vi "PPG_ABC.ProcCases.vi"(0 "i ref in":refnum<vi>, 1 "selector":string, 2 "Data":T1, 3 "call cluster":T2={"Object"="", "Selector"="", "CallType"=enum."synchronous", "Async Object"="", "Async Selector"="", "Data Descriptor"="", "Data"=[], "Error #"=0, "Expire"=0}, 5 "error in (no error)":errorcluster) -> (14 "i ref out":refnum<vi>, 17 "answer cluster":T2={"Object"="", "Selector"="", "CallType"=enum."synchronous", "Async Object"="", "Async Selector"="", "Data Descriptor"="", "Data"=[], "Error #"=0, "Expire"=0}, 19 "error out":errorcluster)   [LabVIEW 2014, in "PPG_ABC.lvlib"]
doc: "This method is called by a process from within the default case in the event loop. The methods of a class that are linked to events will be called from THIS method. Add your code here."
uses:
  PPG_ABC.lvlib
  CSCore/CSSystem/CoreDefs/CoreDefs.call_type.ctl
  CSCore/BaseProcess/BaseProcess.descriptor string definition.ctl
  CSCore/CSSystem/CoreDefs/CoreDefs.rawDataType.ctl
  CSCore/CSSystem/CoreLib/CoreLib.string 2 byte array.vi
  CSCore/CSSystem/CoreLib/CoreLib.byte array 2 int.vi
  CSCore/CSSystem/CoreLib/CoreLib.int 2 byte array.vi
  CSCore/CSSystem/CoreLib/CoreLib.byte array 2 double.vi
  CSCore/CSSystem/CoreLib/CoreLib.byte array 2 string.vi
  CSCore/CSSystem/CoreLib/CoreLib.lvlib
  CSCore/BaseProcess/BaseProcess.lvlib
  NI_FPGA_PPG/NI_FPGA_PPG.lvlib
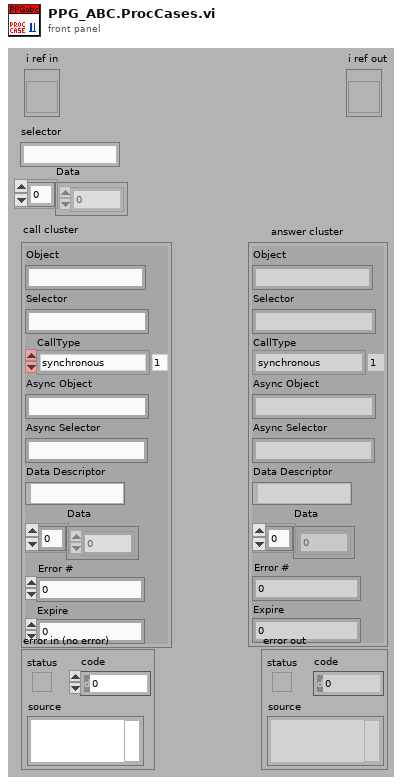
[diagram p1: front panel]
types:
  T1 = typedef "CoreDefs.rawDataType.ctl" = i8[]
  T2 = typedef "CoreDefs.call_type.ctl" = cluster{"Object":string, "Selector":string, "CallType":enum16{"simple", "synchronous", "asynchronous"}, "Async Object":string, "Async Selector":string, "Data Descriptor":T3, "Data":T1, "Error #":i32, "Expire":u32}
  T3 = typedef "BaseProcess.lvlib/BaseProcess.descriptor string definition.ctl" = string
  T4 = typedef "PPG_ABC.lvlib/PPG_ABC.PG_dataType.ctl" = cluster{"PGDevice":string, "rawPatternData":cluster{"triggerCondition":i32, "timeTable":dbl[], "channelTable":string[]}[]}
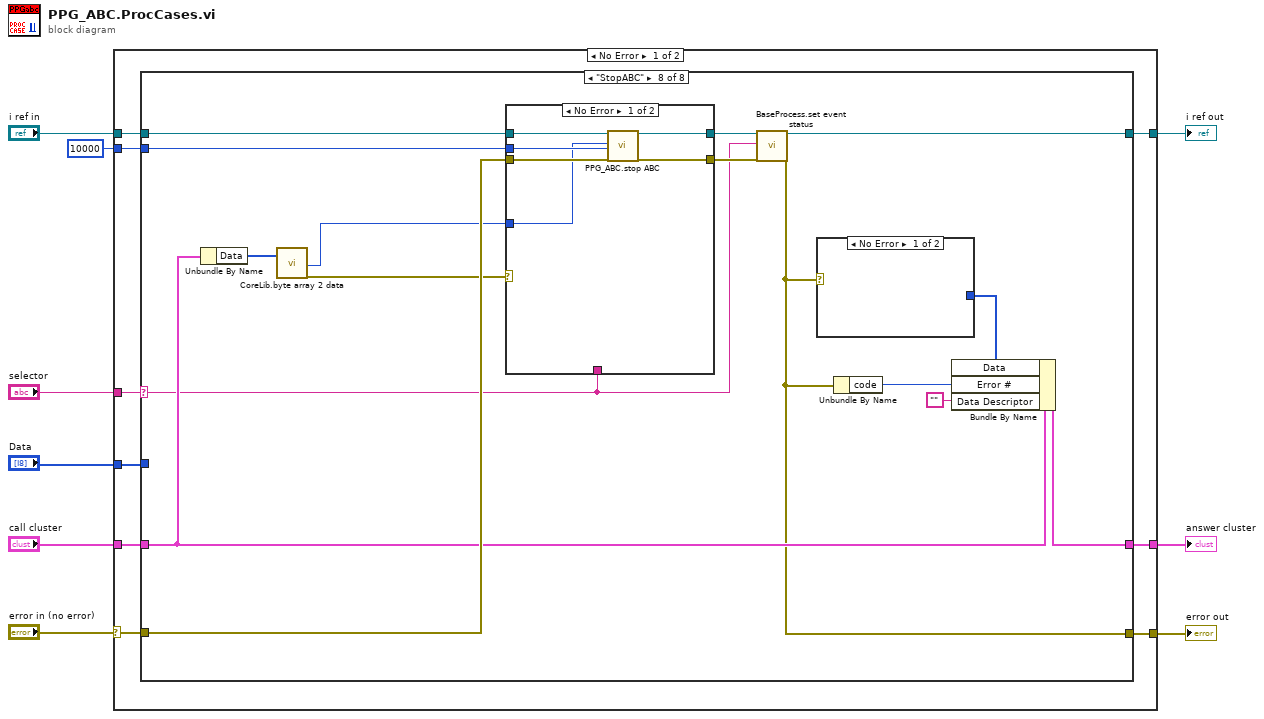
[diagram p0: block diagram]
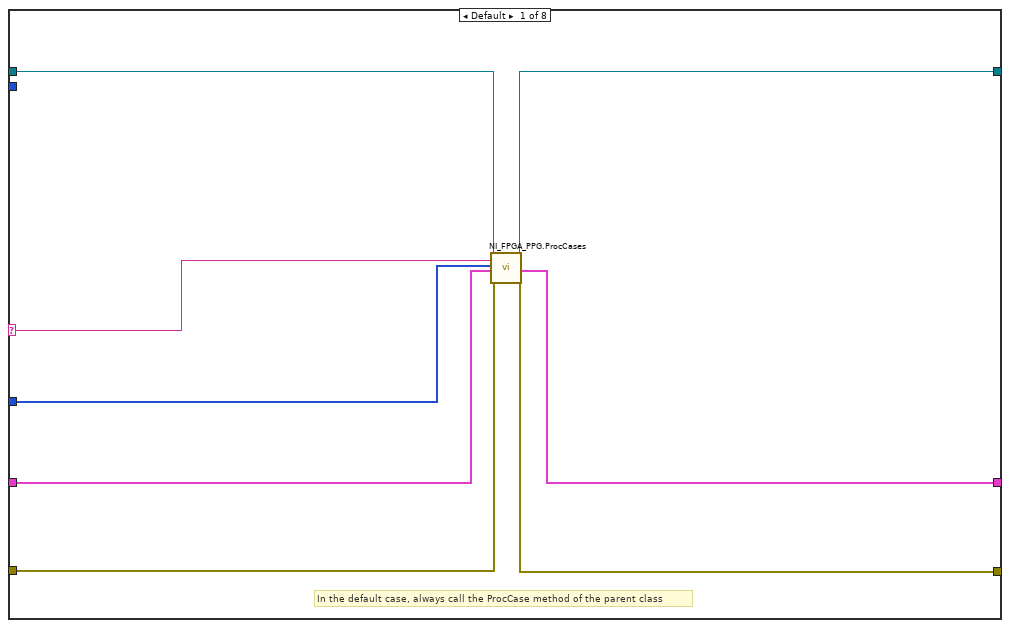
[diagram p2: hidden frame]
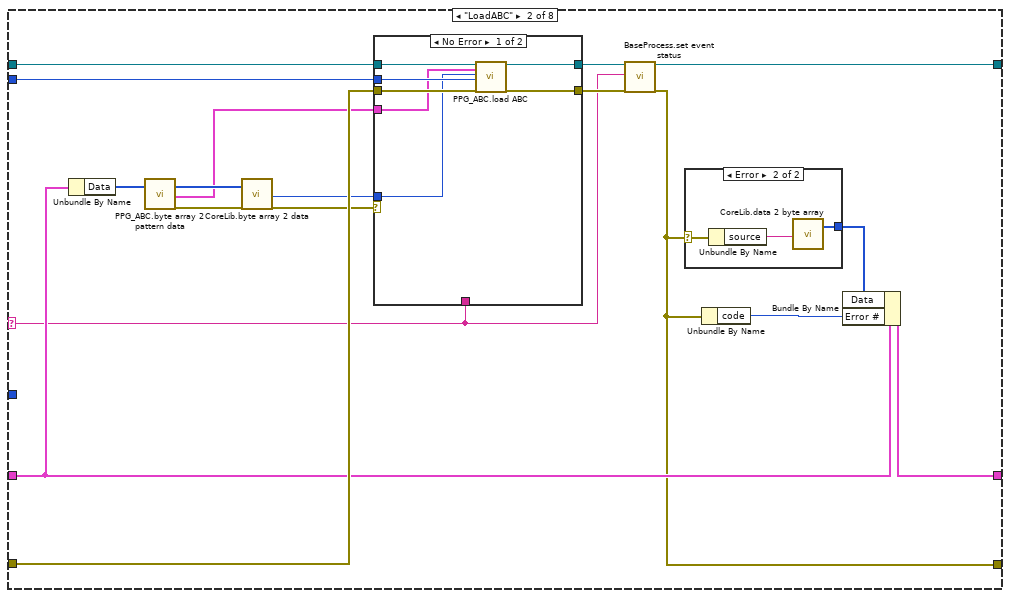
[diagram p3: hidden frame]
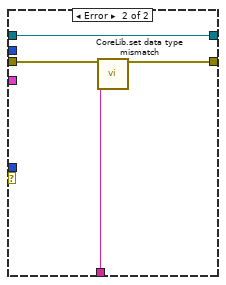
[diagram p5: hidden frame]
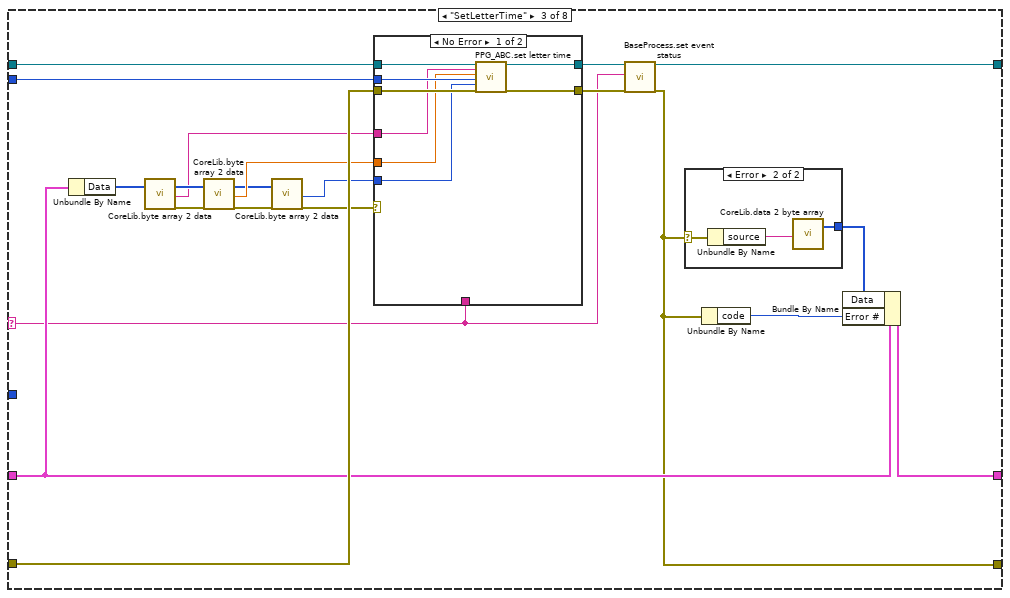
[diagram p6: hidden frame]
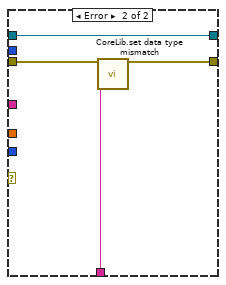
[diagram p8: hidden frame]
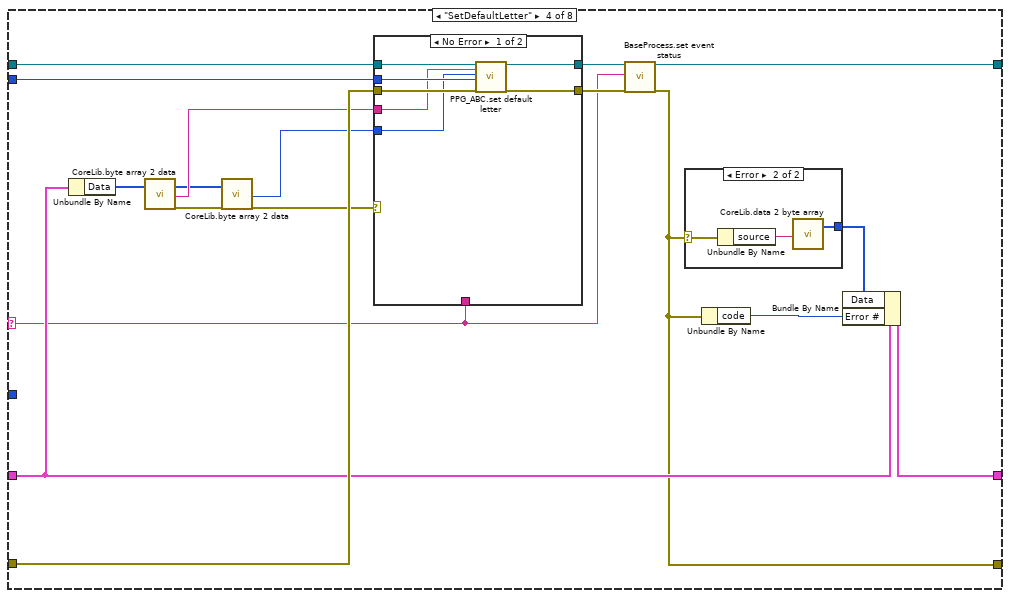
[diagram p9: hidden frame]
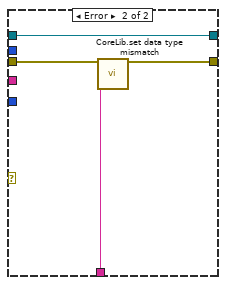
[diagram p11: hidden frame]
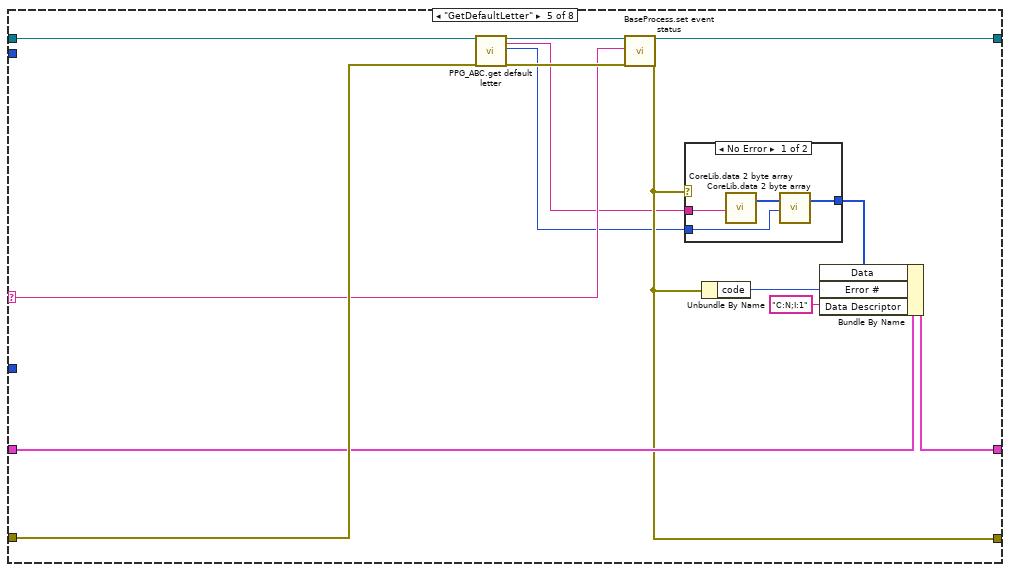
[diagram p12: hidden frame]
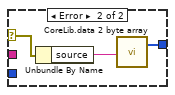
[diagram p13: hidden frame]
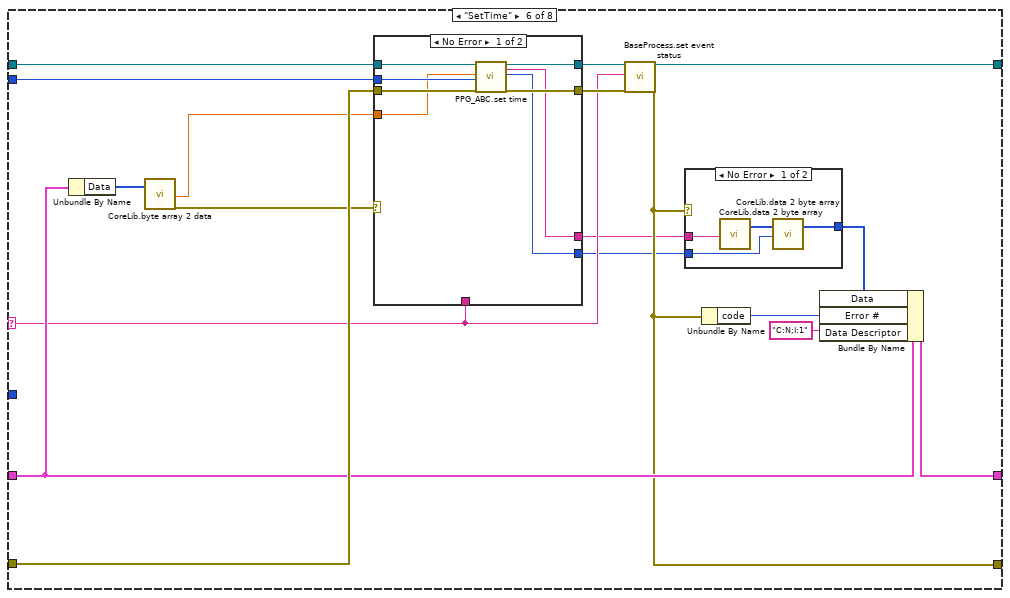
[diagram p14: hidden frame]
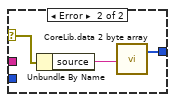
[diagram p15: hidden frame]
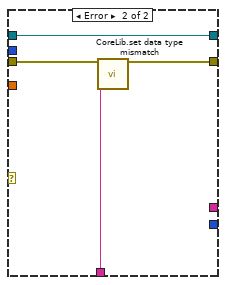
[diagram p16: hidden frame]
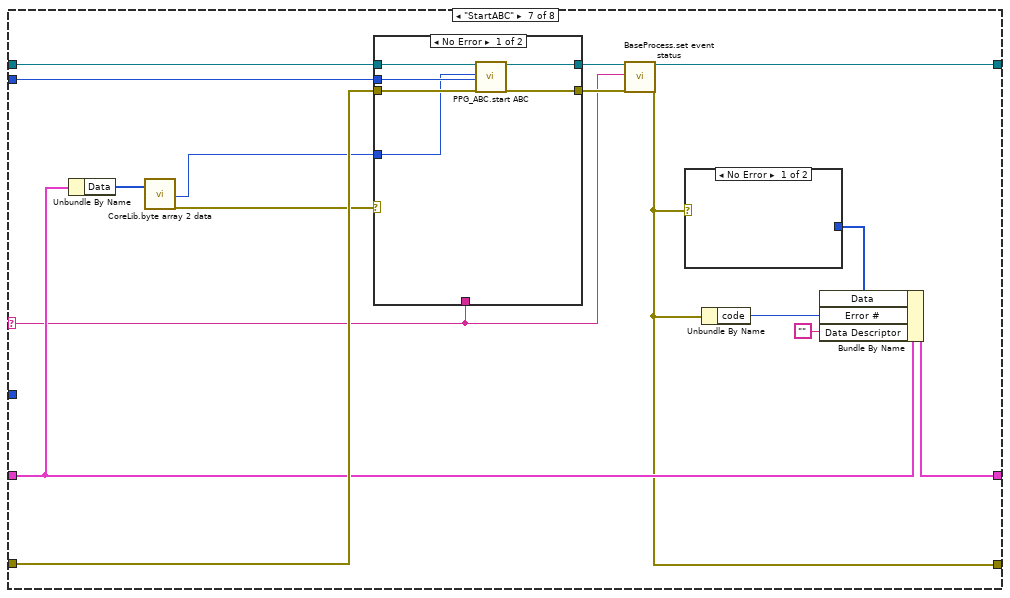
[diagram p17: hidden frame]
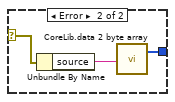
[diagram p18: hidden frame]
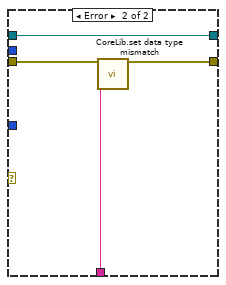
[diagram p19: hidden frame]
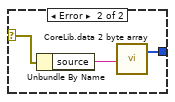
[diagram p20: hidden frame]
diagram:
  n1 = case shown="No Error" "error in (no error)" {
    selector: "error in (no error)" -> [w11 w243]
    tunnel: "selector" -> [w18 _]
    tunnel: [w17 w244] -> w8
    tunnel: "Data" -> [w16 _]
    tunnel: "call cluster" -> [w15 w244]
    tunnel: "i ref in" -> [w14 w245]
    tunnel: [w13 w245] -> w4
    tunnel: [w12 w243] -> w3
    tunnel: 10000 ("ms timeout [ms]") -> [w10 _]
    frame No Error {
      n2 = case shown="\"StopABC\"" w18 {
        selector: w18 -> [w21 w35 w70 w103 w131 w156 w191 w220]
        tunnel: w16 -> [w19 _ _ _ _ _ _ _]
        tunnel: w14 -> [w20 w44 w79 w112 w140 w165 w200 w229]
        tunnel: [w26 w34 w69 w102 w130 w155 w190 w219] -> w13
        tunnel: w15 -> [w22 w41 w76 w109 w137 w162 w197 w226]
        tunnel: [w23 w40 w75 w108 w136 w161 w196 w225] -> w17
        tunnel: w11 -> [w25 w43 w78 w111 w139 w164 w199 w228]
        tunnel: [w24 w36 w71 w104 w132 w157 w192 w221] -> w12
        tunnel: w10 -> [_ w32 w67 w100 _ w153 w188 w217]
        frame Default {
          # "In the default case, always call the ProcCase method of the parent class"
          n3 = call "NI_FPGA_PPG.ProcCases.vi"("i ref in"=w20, "selector"=w21, "Data"=w19, "call cluster"=w22, "error in (no error)"=w25) -> ("i ref out"=w26:refnum<vi>, "answer cluster"=w23:T2, "error out"=w24:errorcluster)  [unwired: 12 in]
        }
        frame "LoadABC" {
          n4 = Unbundle By Name(w41) -> ("Data"=w33:T1)
          n5 = call "PPG_ABC.byte array 2 pattern data.vi"("byteArray"=w33) -> ("byteArray out"=w29:T1, "PGData out"=w28:T4, "error out"=w31:errorcluster)  [unwired: 16 in]
          n6 = call-poly "CoreLib.byte array 2 data.vi"("byteArray"=w29, "error in (no error)"=w31) -> ("i32"=w27:i32, "error out"=w30:errorcluster)  [unwired: 15 in, 1 out]
          n7 = case shown="No Error" w30 {
            tunnel: [w51 w58] -> w38
            tunnel: w44 -> [w54 w58]
            tunnel: w43 -> [w53 w57]
            tunnel: [w50 w56] -> w37
            tunnel: w35 -> [_ w55]
            tunnel: w32 -> [w52 _]
            tunnel: w28 -> [w49 _]
            tunnel: w27 -> [w48 _]
            frame No Error {
              n8 = call "PPG_ABC.load ABC.vi"("i ref in"=w54, "PGData"=w49, "patternGroup"=w48, "ms timeout [ms]"=w52, "error in (no error)"=w53) -> ("i ref out"=w51:refnum<vi>, "error out"=w50:errorcluster)  [unwired: 12 in, 1 out]
            }
            frame Error {
              n9 = call "CoreLib.set data type mismatch.vi"("error in (no error)"=w57, "error source"=w55) -> ("error out"=w56:errorcluster)  [unwired: 17 in]
            }
          }
          n10 = call "BaseProcess.set event status.vi"("i ref in"=w38, "EventStatus"=w35, "error in (no error)"=w37) -> ("i ref out"=w34:refnum<vi>, "error out"=w36:errorcluster)  [unwired: 14 in, 1 out]
          n11 = case shown="Error" w36 {
            selector: w36 -> [_ w47]
            tunnel: [_ w46] -> w39
            frame No Error {
            }
            frame Error {
              n12 = Unbundle By Name(w47) -> ("source"=w45:string)
              n13 = call-poly "CoreLib.data 2 byte array.vi"("string"=w45) -> ("byteArray out"=w46:T1)  [unwired: 18 in]
            }
          }
          n14 = Unbundle By Name(w36) -> ("code"=w42:i32)
          n15 = Bundle By Name(cluster=w41, "Data"=w39, "Error #"=w42) -> (w40:T2)
        }
        frame "SetLetterTime" {
          n16 = Unbundle By Name(w76) -> ("Data"=w68:T1)
          n17 = call-poly "CoreLib.byte array 2 data.vi"("byteArray"=w68) -> ("byteArray out"=w66:T1, "string"=w64:string, "error out"=w65:errorcluster)  [unwired: 16 in]
          n18 = call-poly "CoreLib.byte array 2 data.vi"("byteArray"=w66, "error in (no error)"=w65) -> ("byteArray out"=w60:T1, "d64"=w63:dbl, "error out"=w62:errorcluster)  [unwired: 15 in]
          n19 = call-poly "CoreLib.byte array 2 data.vi"("byteArray"=w60, "error in (no error)"=w62) -> ("i32"=w59:i32, "error out"=w61:errorcluster)  [unwired: 15 in, 1 out]
          n20 = case shown="No Error" w61 {
            tunnel: [w87 w94] -> w73
            tunnel: w79 -> [w90 w94]
            tunnel: w78 -> [w89 w93]
            tunnel: [w86 w92] -> w72
            tunnel: w70 -> [_ w91]
            tunnel: w67 -> [w88 _]
            tunnel: w64 -> [w85 _]
            tunnel: w63 -> [w84 _]
            tunnel: w59 -> [w83 _]
            frame No Error {
              n21 = call "PPG_ABC.set letter time.vi"("i ref in"=w90, "letter"=w85, "time [us]"=w84, "ms timeout [ms]"=w88, "patternGroup"=w83, "error in (no error)"=w89) -> ("i ref out"=w87:refnum<vi>, "error out"=w86:errorcluster)  [unwired: 11 in, 1 out]
            }
            frame Error {
              n22 = call "CoreLib.set data type mismatch.vi"("error in (no error)"=w93, "error source"=w91) -> ("error out"=w92:errorcluster)  [unwired: 17 in]
            }
          }
          n23 = call "BaseProcess.set event status.vi"("i ref in"=w73, "EventStatus"=w70, "error in (no error)"=w72) -> ("i ref out"=w69:refnum<vi>, "error out"=w71:errorcluster)  [unwired: 14 in, 1 out]
          n24 = case shown="Error" w71 {
            selector: w71 -> [_ w82]
            tunnel: [_ w81] -> w74
            frame No Error {
            }
            frame Error {
              n25 = Unbundle By Name(w82) -> ("source"=w80:string)
              n26 = call-poly "CoreLib.data 2 byte array.vi"("string"=w80) -> ("byteArray out"=w81:T1)  [unwired: 18 in]
            }
          }
          n27 = Unbundle By Name(w71) -> ("code"=w77:i32)
          n28 = Bundle By Name(cluster=w76, "Data"=w74, "Error #"=w77) -> (w75:T2)
        }
        frame "SetDefaultLetter" {
          n29 = Unbundle By Name(w109) -> ("Data"=w101:T1)
          n30 = call-poly "CoreLib.byte array 2 data.vi"("byteArray"=w101) -> ("byteArray out"=w96:T1, "string"=w99:string, "error out"=w98:errorcluster)  [unwired: 16 in]
          n31 = call-poly "CoreLib.byte array 2 data.vi"("byteArray"=w96, "error in (no error)"=w98) -> ("i32"=w95:i32, "error out"=w97:errorcluster)  [unwired: 15 in, 1 out]
          n32 = case shown="No Error" w97 {
            tunnel: [w119 w126] -> w106
            tunnel: w112 -> [w122 w126]
            tunnel: w111 -> [w121 w125]
            tunnel: [w118 w124] -> w105
            tunnel: w103 -> [_ w123]
            tunnel: w100 -> [w120 _]
            tunnel: w99 -> [w117 _]
            tunnel: w95 -> [w116 _]
            frame No Error {
              n33 = call "PPG_ABC.set default letter.vi"("i ref in"=w122, "letter"=w117, "patternGroup"=w116, "ms timeout [ms]"=w120, "error in (no error)"=w121) -> ("i ref out"=w119:refnum<vi>, "error out"=w118:errorcluster)  [unwired: 12 in, 1 out]
            }
            frame Error {
              n34 = call "CoreLib.set data type mismatch.vi"("error in (no error)"=w125, "error source"=w123) -> ("error out"=w124:errorcluster)  [unwired: 17 in]
            }
          }
          n35 = call "BaseProcess.set event status.vi"("i ref in"=w106, "EventStatus"=w103, "error in (no error)"=w105) -> ("i ref out"=w102:refnum<vi>, "error out"=w104:errorcluster)  [unwired: 14 in, 1 out]
          n36 = case shown="Error" w104 {
            selector: w104 -> [_ w115]
            tunnel: [_ w114] -> w107
            frame No Error {
            }
            frame Error {
              n37 = Unbundle By Name(w115) -> ("source"=w113:string)
              n38 = call-poly "CoreLib.data 2 byte array.vi"("string"=w113) -> ("byteArray out"=w114:T1)  [unwired: 18 in]
            }
          }
          n39 = Unbundle By Name(w104) -> ("code"=w110:i32)
          n40 = Bundle By Name(cluster=w109, "Data"=w107, "Error #"=w110) -> (w108:T2)
        }
        frame "GetDefaultLetter" {
          n41 = call "PPG_ABC.get default letter.vi"("i ref in"=w140, "error in (no error)"=w139) -> ("i ref out"=w134:refnum<vi>, "letter"=w128:string, "patternGroup"=w127:i32, "error out"=w133:errorcluster)  [unwired: 14 in]
          n42 = call "BaseProcess.set event status.vi"("i ref in"=w134, "EventStatus"=w131, "error in (no error)"=w133) -> ("i ref out"=w130:refnum<vi>, "error out"=w132:errorcluster)  [unwired: 14 in, 1 out]
          n43 = case shown="No Error" w132 {
            selector: w132 -> [_ w147]
            tunnel: [w142 w146] -> w135
            tunnel: w128 -> [w144 _]
            tunnel: w127 -> [w141 _]
            frame No Error {
              n44 = call-poly "CoreLib.data 2 byte array.vi"("string"=w144) -> ("byteArray out"=w143:T1)  [unwired: 18 in]
              n45 = call-poly "CoreLib.data 2 byte array.vi"("byteArray"=w143, "i32"=w141) -> ("byteArray out"=w142:T1)  [unwired: 17 in]
            }
            frame Error {
              n46 = Unbundle By Name(w147) -> ("source"=w145:string)
              n47 = call-poly "CoreLib.data 2 byte array.vi"("string"=w145) -> ("byteArray out"=w146:T1)  [unwired: 18 in]
            }
          }
          n48 = Unbundle By Name(w132) -> ("code"=w138:i32)
          n49 = Bundle By Name(cluster=w137, "Data"=w135, "Error #"=w138, "Data Descriptor"=T3 "C:N;I:1") -> (w136:T2)
        }
        frame "SetTime" {
          n50 = Unbundle By Name(w162) -> ("Data"=w154:T1)
          n51 = call-poly "CoreLib.byte array 2 data.vi"("byteArray"=w154) -> ("d64"=w152:dbl, "error out"=w151:errorcluster)  [unwired: 16 in, 1 out]
          n52 = case shown="No Error" w151 {
            tunnel: [w177 w184] -> w159
            tunnel: w165 -> [w180 w184]
            tunnel: w164 -> [w179 w183]
            tunnel: [w176 w182] -> w158
            tunnel: w156 -> [_ w181]
            tunnel: w153 -> [w178 _]
            tunnel: w152 -> [w175 _]
            tunnel: [w174 _] -> w150
            tunnel: [w173 _] -> w148
            frame No Error {
              n53 = call "PPG_ABC.set time.vi"("i ref in"=w180, "time [us]"=w175, "ms timeout [ms]"=w178, "error in (no error)"=w179) -> ("i ref out"=w177:refnum<vi>, "defaultLetter"=w173:string, "patternGroup"=w174:i32, "error out"=w176:errorcluster)  [unwired: 11 in, 1 out]
            }
            frame Error {
              n54 = call "CoreLib.set data type mismatch.vi"("error in (no error)"=w183, "error source"=w181) -> ("error out"=w182:errorcluster)  [unwired: 17 in]
            }
          }
          n55 = call "BaseProcess.set event status.vi"("i ref in"=w159, "EventStatus"=w156, "error in (no error)"=w158) -> ("i ref out"=w155:refnum<vi>, "error out"=w157:errorcluster)  [unwired: 14 in, 1 out]
          n56 = case shown="No Error" w157 {
            selector: w157 -> [_ w172]
            tunnel: [w169 w171] -> w160
            tunnel: w150 -> [w167 _]
            tunnel: w148 -> [w166 _]
            frame No Error {
              n57 = call-poly "CoreLib.data 2 byte array.vi"("string"=w166) -> ("byteArray out"=w168:T1)  [unwired: 18 in]
              n58 = call-poly "CoreLib.data 2 byte array.vi"("byteArray"=w168, "i32"=w167) -> ("byteArray out"=w169:T1)  [unwired: 17 in]
            }
            frame Error {
              n59 = Unbundle By Name(w172) -> ("source"=w170:string)
              n60 = call-poly "CoreLib.data 2 byte array.vi"("string"=w170) -> ("byteArray out"=w171:T1)  [unwired: 18 in]
            }
          }
          n61 = Unbundle By Name(w157) -> ("code"=w163:i32)
          n62 = Bundle By Name(cluster=w162, "Data"=w160, "Error #"=w163, "Data Descriptor"=T3 "C:N;I:1") -> (w161:T2)
        }
        frame "StartABC" {
          n63 = Unbundle By Name(w197) -> ("Data"=w189:T1)
          n64 = call-poly "CoreLib.byte array 2 data.vi"("byteArray"=w189) -> ("i32"=w187:i32, "error out"=w186:errorcluster)  [unwired: 16 in, 1 out]
          n65 = case shown="No Error" w186 {
            tunnel: [w207 w213] -> w194
            tunnel: w200 -> [w209 w213]
            tunnel: w199 -> [w208 w212]
            tunnel: [w206 w211] -> w193
            tunnel: w191 -> [_ w210]
            tunnel: w188 -> [w205 _]
            tunnel: w187 -> [w204 _]
            frame No Error {
              n66 = call "PPG_ABC.start ABC.vi"("i ref in"=w209, "patternGroup"=w204, "ms timeout [ms]"=w205, "error in (no error)"=w208) -> ("i ref out"=w207:refnum<vi>, "error out"=w206:errorcluster)  [unwired: 13 in, 1 out]
            }
            frame Error {
              n67 = call "CoreLib.set data type mismatch.vi"("error in (no error)"=w212, "error source"=w210) -> ("error out"=w211:errorcluster)  [unwired: 17 in]
            }
          }
          n68 = call "BaseProcess.set event status.vi"("i ref in"=w194, "EventStatus"=w191, "error in (no error)"=w193) -> ("i ref out"=w190:refnum<vi>, "error out"=w192:errorcluster)  [unwired: 14 in, 1 out]
          n69 = case shown="No Error" w192 {
            selector: w192 -> [_ w203]
            tunnel: [_ w202] -> w195
            frame No Error {
            }
            frame Error {
              n70 = Unbundle By Name(w203) -> ("source"=w201:string)
              n71 = call-poly "CoreLib.data 2 byte array.vi"("string"=w201) -> ("byteArray out"=w202:T1)  [unwired: 18 in]
            }
          }
          n72 = Unbundle By Name(w192) -> ("code"=w198:i32)
          n73 = Bundle By Name(cluster=w197, "Data"=w195, "Error #"=w198, "Data Descriptor"="") -> (w196:T2)
        }
        frame "StopABC" {
          n74 = Unbundle By Name(w226) -> ("Data"=w218:T1)
          n75 = call-poly "CoreLib.byte array 2 data.vi"("byteArray"=w218) -> ("i32"=w216:i32, "error out"=w215:errorcluster)  [unwired: 16 in, 1 out]
          n76 = case shown="No Error" w215 {
            tunnel: [w236 w242] -> w223
            tunnel: w229 -> [w238 w242]
            tunnel: w228 -> [w237 w241]
            tunnel: [w235 w240] -> w222
            tunnel: w220 -> [_ w239]
            tunnel: w217 -> [w234 _]
            tunnel: w216 -> [w233 _]
            frame No Error {
              n77 = call "PPG_ABC.stop ABC.vi"("i ref in"=w238, "patternGroup"=w233, "ms timeout [ms]"=w234, "error in (no error)"=w237) -> ("i ref out"=w236:refnum<vi>, "error out"=w235:errorcluster)  [unwired: 13 in, 1 out]
            }
            frame Error {
              n78 = call "CoreLib.set data type mismatch.vi"("error in (no error)"=w241, "error source"=w239) -> ("error out"=w240:errorcluster)  [unwired: 17 in]
            }
          }
          n79 = call "BaseProcess.set event status.vi"("i ref in"=w223, "EventStatus"=w220, "error in (no error)"=w222) -> ("i ref out"=w219:refnum<vi>, "error out"=w221:errorcluster)  [unwired: 14 in, 1 out]
          n80 = case shown="No Error" w221 {
            selector: w221 -> [_ w232]
            tunnel: [_ w231] -> w224
            frame No Error {
            }
            frame Error {
              n81 = Unbundle By Name(w232) -> ("source"=w230:string)
              n82 = call-poly "CoreLib.data 2 byte array.vi"("string"=w230) -> ("byteArray out"=w231:T1)  [unwired: 18 in]
            }
          }
          n83 = Unbundle By Name(w221) -> ("code"=w227:i32)
          n84 = Bundle By Name(cluster=w226, "Data"=w224, "Error #"=w227, "Data Descriptor"="") -> (w225:T2)
        }
      }
    }
    frame Error {
    }
  }
  "answer cluster" <- w8
  "i ref out" <- w4
  "error out" <- w3
